vi "合并单元格.vi"(5 "合并选项":enum16{"合并", "按行合并", "取消合并"}(ring), 7 "工作表名称":string="Sheet1", 8 "错误输入（无错误）":errorcluster, 11 "单元格区域":T1={"起始列"="A", "起始行"=1, "大小"=[]} {"大小" min=1 max=1048576; "起始行" min=1 max=1048576}) -> (0 "错误输出":errorcluster)   [LabVIEW 2020, in "OperateExcel.lvlib"]
uses:
  OperateExcel.lvlib
  Globals.vi
  <vilib>/Utility/error.llb/Error Cluster From Error Code.vi
  <vilib>/ErrorRing/Error Ring.xnode
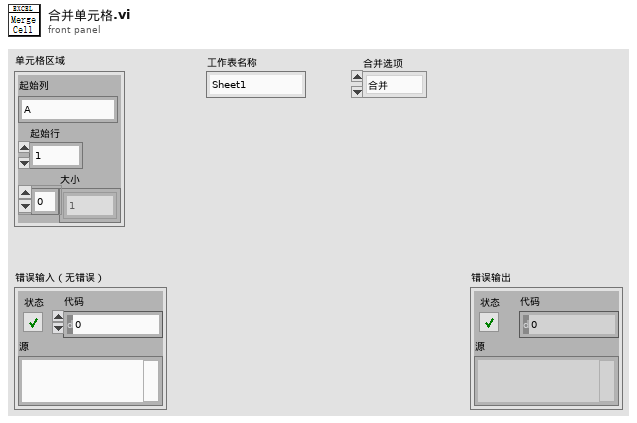
[diagram p1: front panel]
types:
  T1 = typedef "OperateExcel.lvlib/单元格区域.ctl" = cluster{"起始列":string, "起始行":u32, "大小":u32[]}
  T2 = typedef "OperateExcel.lvlib/引用簇.ctl" = cluster{"Excel._Application":refnum<k7>, "Workbooks":refnum<k7>, "Open":refnum<k7>, "Worksheets":refnum<k7>, "sheetList":refnum<k7>[]}
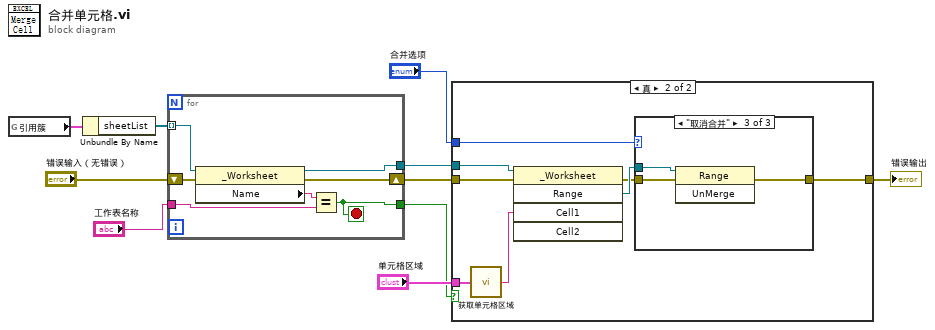
[diagram p0: block diagram]
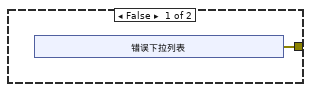
[diagram p2: hidden frame]
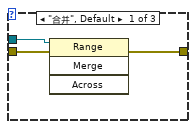
[diagram p3: hidden frame]
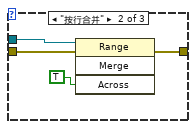
[diagram p4: hidden frame]
diagram:
  n1 = global read "Globals.vi" "引用簇"() -> (w3:T2)
  n2 = Unbundle By Name(w3) -> ("sheetList"=w10:refnum<k7>[])
  n3 = for {
    tunnel: w10 -> [w17] mode=indexing
    tunnel: "工作表名称" -> [w15]
    tunnel: [w14] -> w9
    shift-right: [w12] -> w7
    shift-left: "错误输入（无错误）" -> [w13]
    tunnel: [w11] -> w1
    stop <- w11 stop-if-true
    n4 = property class="_Worksheet"(reference=w17, error in=w13) -> (reference out=w14:refnum<k7>, error out=w12:errorcluster, "Name"=w16:string)
    n5 = Equal?(x=w16, y=w15) -> (x = y?=w11:bool)
  }
  n6 = case shown="真" w1 {
    tunnel: w9 -> [_ w30]
    tunnel: w7 -> [_ w29]
    tunnel: [w18 w26] -> w6
    tunnel: "单元格区域" -> [_ w24]
    tunnel: "合并选项" -> [_ w23]
    frame False {
      n7 = xnode "错误下拉列表"() -> ("错误输出"=w18:errorcluster)
    }
    frame True {
      n8 = call "获取单元格区域.vi"("单元格区域"=w24) -> ("单元格区域"=w25:string)
      n9 = invoke class="_Worksheet" method="Range"(reference=w30, error in=w29, "Cell1"=w25) -> (error out=w27:errorcluster, "Range"=w28:refnum<k7>)  [unwired: 2 in, 3 out]
      n10 = case shown="\"取消合并\"" w23 {
        tunnel: w28 -> [w33 w37 w40]
        tunnel: w27 -> [w32 w36 w39]
        tunnel: [w31 w35 w38] -> w26
        frame "合并", Default {
          n11 = invoke on="调用节点" class="Range" method="Merge"(reference=w33, error in=w32) -> (error out=w31:errorcluster)  [unwired: 2 in, 3 out]
        }
        frame "按行合并" {
          n12 = invoke on="调用节点" class="Range" method="Merge"(reference=w37, error in=w36, "Across"=TRUE) -> (error out=w35:errorcluster)  [unwired: 1 in, 3 out]
        }
        frame "取消合并" {
          n13 = invoke on="调用节点" class="Range" method="UnMerge"(reference=w40, error in=w39) -> (error out=w38:errorcluster)  [unwired: 1 in, 2 out]
        }
      }
    }
  }
  "错误输出" <- w6
